vi "UDT_programControlModule_PostRunCTRL.vi"() -> (3 "Unit Test Framework Results":T1)   [LabVIEW 2017]
doc: "Use this template to create a user-defined test VI. Define your test requirements and wire the results to the <b>Result (Test)</b> control. Do not modify the <b>Unit Test Framework Results</b> indicator."
uses:
  <vilib>/utf/common/utf_test_result_troll.ctl
  <vilib>/utf/common/utf_test_result.ctl
  <vilib>/utf/common/utf_test_result_failure.ctl
  <vilib>/utf/common/utf_test_comparison_operators.ctl
  <vilib>/utf/common/utf_vi_tag.ctl
  RT/programControl/Queue/TypeDefs/queueFGVState.ctl
  RT/programControl/Queue/TypeDefs/message.ctl
  RT/programControl/StartUEFGV/TypeDefs/UEFGVcontrol.ctl
  <vilib>/Control Software Solutions Ltd/UTF Helper/SubVIs/UTF Variant Equals.vi
  <vilib>/Control Software Solutions Ltd/UTF Helper/Unit Test Helper.lvlib
  RT/programControl/programControl.lvlib
  <vilib>/utf/NI_UnitTestFramework.lvlib
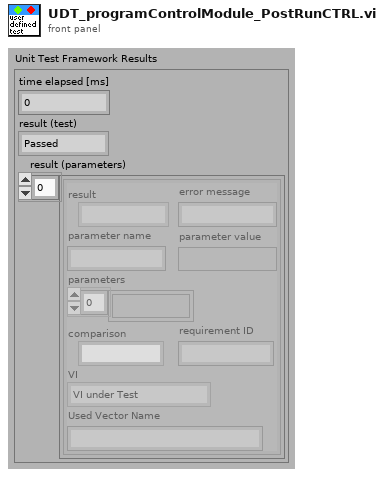
[diagram p1: front panel]
types:
  T1 = typedef "NI_UnitTestFramework.lvlib/utf_test_result_troll.ctl" = cluster{"time elapsed [ms]":u32, "result (test)":T2, "result (parameters)":T3[]}
  T2 = typedef "NI_UnitTestFramework.lvlib/utf_test_result.ctl" = enum16{"Passed", "Failed", "Error", "Skipped", "Not Processed"}
  T3 = typedef "NI_UnitTestFramework.lvlib/utf_test_result_failure.ctl" = cluster{"result":T2, "error message":string, "parameter name":string, "parameter value":variant, "parameters":variant[], "comparison":T4, "requirement ID":string, "VI":T5, "Used Vector Name":string}
  T4 = typedef "NI_UnitTestFramework.lvlib/utf_test_comparison_operators.ctl" = enum16{"=", "!=", ">", ">=", "<", "<=", "range", "symmetric tolerance", "asymmetric tolerance", "string contains", "string not contain", "array size", "string length", "array range", "by element", "array range (limit array)", "user-defined", "array contains", "array not contain", "vector length", "= (elm)", "!= (elm)", "= (case insensitive)", "!= (case insensitive)"}
  T5 = typedef "NI_UnitTestFramework.lvlib/utf_vi_tag.ctl" = enum16{"Setup VI", "VI under Test", "Teardown VI"}
  T6 = typedef "UEFGVcontrol.ctl" = enum16{"Create", "Get", "Destroy"}
  T7 = typedef "programControl.lvlib/message.ctl" = cluster{"calling module":string, "message":string, "Data":variant}
  T8 = typedef "programControl.lvlib/queueFGVState.ctl" = enum16{"obtain", "enqueue (low priority)", "enqueue (high priority)", "dequeue", "release"}
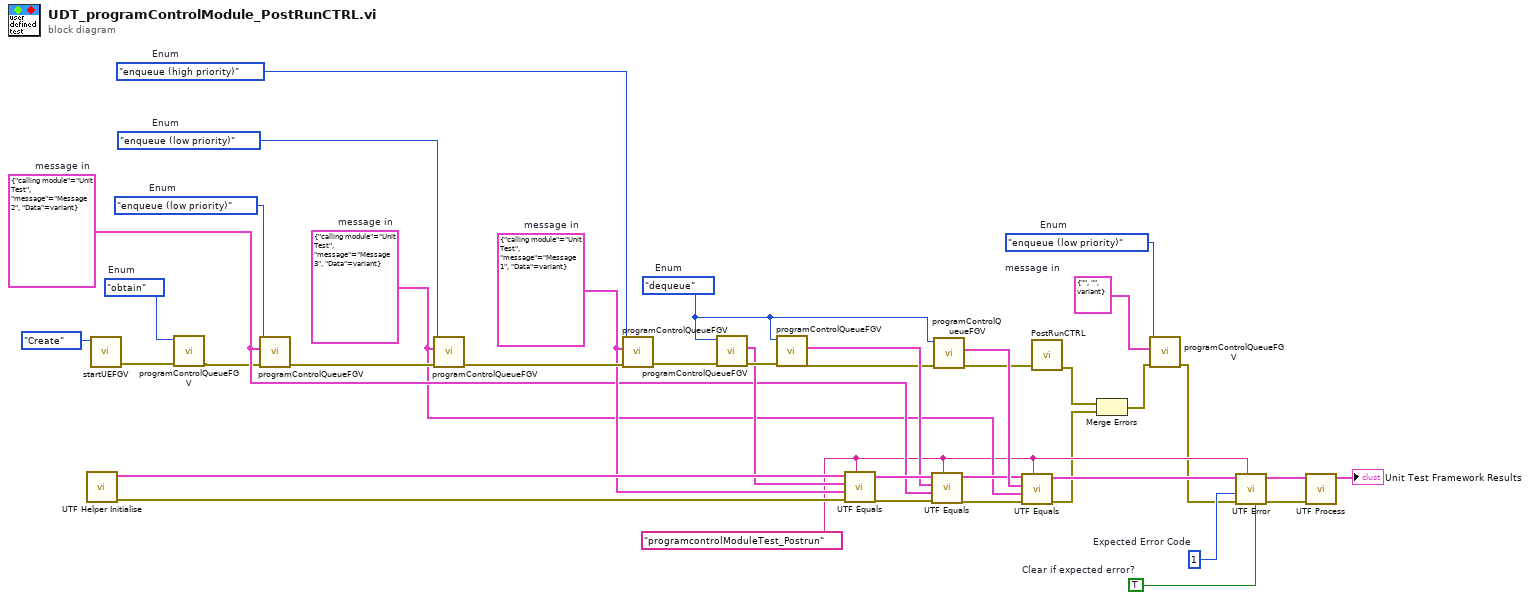
[diagram p0: block diagram]
diagram:
  w8 = TRUE  # Clear if expected error?
  w9 = 1  # Expected Error Code
  w14 = T7 {"calling module"="", "message"="", "Data"=variant}  # message in
  w15 = queueFGVState."enqueue (low priority)"  # Enum
  w17 = queueFGVState."obtain"  # Enum
  w10 = "programcontrolModuleTest_Postrun"
  w24 = queueFGVState."dequeue"  # Enum
  w33 = T7 {"calling module"="Unit Test", "message"="Message 1", "Data"=variant}  # message in
  w20 = T7 {"calling module"="Unit Test", "message"="Message 3", "Data"=variant}  # message in
  w26 = T7 {"calling module"="Unit Test", "message"="Message 2", "Data"=variant}  # message in
  w36 = queueFGVState."enqueue (high priority)"  # Enum
  w38 = queueFGVState."enqueue (low priority)"  # Enum
  w39 = queueFGVState."enqueue (low priority)"  # Enum
  n1 = call <vilib>:"UTF Helper Initialise.vi"() -> ("error out"=w19:errorcluster, "results array"=w34:T3[])  [unwired: 10 in]
  n2 = call "startUEFGV.vi"("Enum"=UEFGVcontrol."Create") -> ("error out"=w2:errorcluster)  [unwired: 9 in, 1 out]
  n3 = call "programControlQueueFGV.vi"("error in (no error)"=w2, "Enum"=w17) -> ("error out"=w18:errorcluster)  [unwired: 8 in, 1 out]
  n4 = call "programControlQueueFGV.vi"("error in (no error)"=w18, "message in"=w26, "Enum"=w39) -> ("error out"=w37:errorcluster)  [unwired: 7 in, 1 out]
  n5 = call "programControlQueueFGV.vi"("error in (no error)"=w37, "message in"=w20, "Enum"=w38) -> ("error out"=w35:errorcluster)  [unwired: 7 in, 1 out]
  n6 = call "programControlQueueFGV.vi"("error in (no error)"=w35, "message in"=w33, "Enum"=w36) -> ("error out"=w32:errorcluster)  [unwired: 7 in, 1 out]
  n7 = call "programControlQueueFGV.vi"("error in (no error)"=w32, "Enum"=w24) -> ("error out"=w29:errorcluster, "message out"=w28:T7)  [unwired: 8 in]
  n8 = call "programControlQueueFGV.vi"("error in (no error)"=w29, "Enum"=w24) -> ("error out"=w25:errorcluster, "message out"=w27:T7)  [unwired: 8 in]
  n9 = call-poly <vilib>:"UTF Equals.vi"("Parameter Name"=w10, "error in (no error)"=w19, "Test Value"=w33, "Input"=w28, "Input Results"=w34) -> ("error out"=w31:errorcluster, "Output Results"=w30:T3[])  [unwired: 5 in]
  n10 = call-poly <vilib>:"UTF Equals.vi"("Parameter Name"=w10, "error in (no error)"=w31, "Test Value"=w26, "Input"=w27, "Input Results"=w30) -> ("error out"=w21:errorcluster, "Output Results"=w22:T3[])  [unwired: 5 in]
  n11 = call "programControlQueueFGV.vi"("error in (no error)"=w25, "Enum"=w24) -> ("error out"=w16:errorcluster, "message out"=w23:T7)  [unwired: 8 in]
  n12 = call-poly <vilib>:"UTF Equals.vi"("Parameter Name"=w10, "error in (no error)"=w21, "Test Value"=w20, "Input"=w23, "Input Results"=w22) -> ("error out"=w6:errorcluster, "Output Results"=w12:T3[])  [unwired: 5 in]
  n13 = call "PostRunCTRL.vi"("error in (no error)"=w16) -> ("error out"=w7:errorcluster)  [unwired: 10 in]
  n14 = Merge Errors(w7, w6) -> (w5:errorcluster)
  n15 = call "programControlQueueFGV.vi"("error in (no error)"=w5, "message in"=w14, "Enum"=w15) -> ("error out"=w4:errorcluster)  [unwired: 7 in, 1 out]
  n16 = call <vilib>:"UTF Error.vi"("Clear if expected error?"=w8, "Parameter Name"=w10, "error in (no error)"=w4, "Expected Error Code"=w9, "Input Results"=w12) -> ("error out"=w13:errorcluster, "Output Results"=w11:T3[])  [unwired: 5 in]
  n17 = call <vilib>:"UTF Process.vi"("error in (no error)"=w13, "results array"=w11) -> ("Unit Test Framework Results"=→"Unit Test Framework Results":T1)  [unwired: 9 in]
